vi "Main.vi"() -> ()   [LabVIEW 2025]
uses:
  TypeDefs/MainState.ctl
  random-number-analyzer-bak/Source/Typedefs/State_enum.ctl
  <vilib>/Analysis/baseanly.llb/Mean (DBL).vi
  <vilib>/Analysis/NI_AALBase.lvlib
  Utilities/Random/Random.lvlib
panel:
  in  "Find Minimum":bool
  in  "Find Maximum":bool
  in  "Compute Average":bool
  in  "Generate Random":bool
  out "Waveform Graph":dbl[](graph)
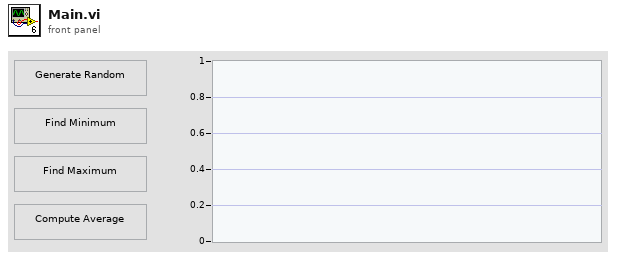
[diagram p1: front panel]
types:
  T1 = typedef "MainState.ctl" = enum16{"CONSTRUCT", "DESTRUCT", "WAITING_FOR_EVENT", "GENERATE_RANDOM", "FIND_MINIMUM", "FIND_MAXIMUM", "COMPUTE_AVERAGE"}
  T2 = typedef "State_enum.ctl" = enum16{"CONSTRUCT", "DESTRUCT", "WAITING_FOR_EVENT", "GENERATE_RANDOM", "FIND_MINIMUM", "FIND_MAXIMUM", "COMPUTE_AVERAGE"}
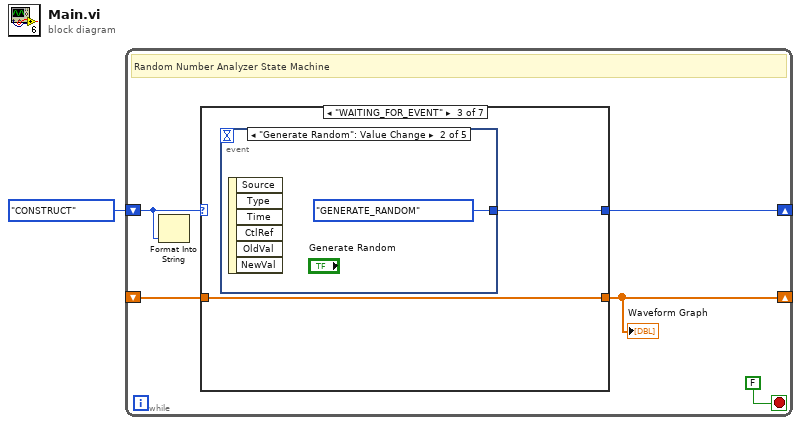
[diagram p0: block diagram]
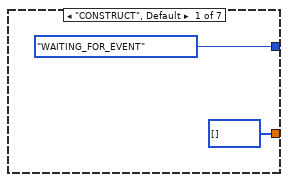
[diagram p2: hidden frame]
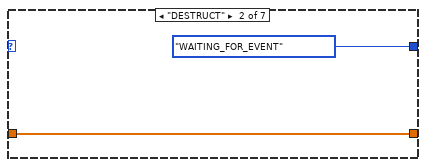
[diagram p3: hidden frame]
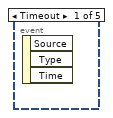
[diagram p4: hidden frame]
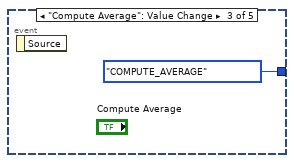
[diagram p5: hidden frame]
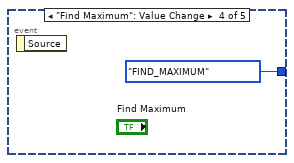
[diagram p6: hidden frame]
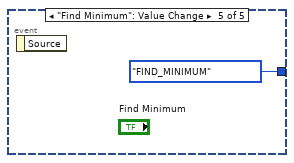
[diagram p7: hidden frame]
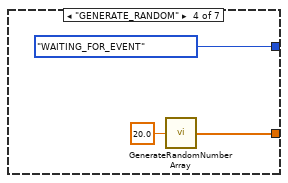
[diagram p8: hidden frame]
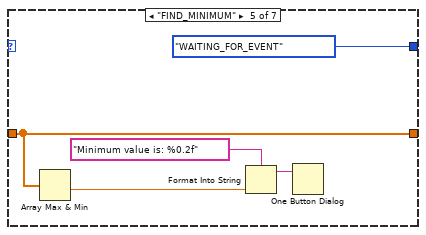
[diagram p9: hidden frame]
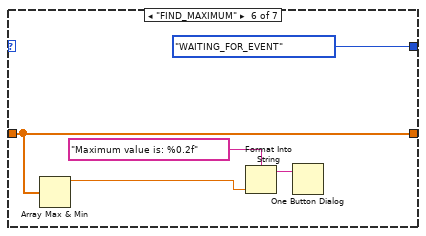
[diagram p10: hidden frame]
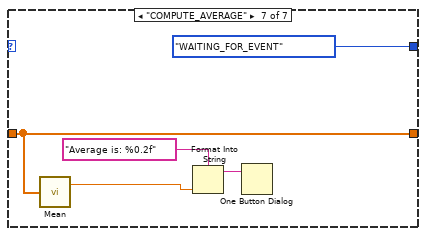
[diagram p11: hidden frame]
diagram:
  n1 = while {
    shift-right: [w5] -> _
    shift-left: MainState."CONSTRUCT" -> [w4]
    shift-right: [w2] -> _
    shift-left: _ -> [w3]
    stop <- FALSE stop-if-true
    # "Random Number Analyzer State Machine"
    n2 = Format Into String(w4) -> ()  [unwired: 3 in, 2 out]
    n3 = case shown="\"WAITING_FOR_EVENT\"" w4 {
      tunnel: [MainState."WAITING_FOR_EVENT" MainState."WAITING_FOR_EVENT" w11 MainState."WAITING_FOR_EVENT" MainState."WAITING_FOR_EVENT" MainState."WAITING_FOR_EVENT" MainState."WAITING_FOR_EVENT"] -> w5
      tunnel: [i32[] [] w10 w12 w17 w23 w25 w33] -> w2
      tunnel: w3 -> [_ w10 w12 _ w23 w25 w33]
      frame "CONSTRUCT", Default {
      }
      frame "DESTRUCT" {
      }
      frame "WAITING_FOR_EVENT" {
        n4 = event shown="[1] \"Generate Random\": Value Change" {
          selector: _ -> [_ _ _ _ _]
          dyn-events: _ -> [_ _ _ _ _]
          timeout: _ -> [_ _ _ _ _]
          tunnel: [_ MainState."GENERATE_RANDOM" State_enum."COMPUTE_AVERAGE" State_enum."FIND_MAXIMUM" State_enum."FIND_MINIMUM"] -> w11
          event Timeout {
            n5 = event-data() -> ()  [unwired: 1 in, 3 out]
          }
          event "Generate Random": Value Change {
            n6 = event-data() -> ()  [unwired: 1 in, 6 out]
          }
          event "Compute Average": Value Change {
            n7 = event-data() -> ()  [unwired: 1 in, 1 out]
          }
          event "Find Maximum": Value Change {
            n8 = event-data() -> ()  [unwired: 1 in, 1 out]
          }
          event "Find Minimum": Value Change {
            n9 = event-data() -> ()  [unwired: 1 in, 1 out]
          }
        }
      }
      frame "GENERATE_RANDOM" {
        n10 = call "GenerateRandomNumberArray.vi"("Size"=20.0) -> ("Array"=w17:dbl[])
      }
      frame "FIND_MINIMUM" {
        n11 = Array Max & Min(array=w23) -> (min value=w20:dbl)  [unwired: 3 out]
        n12 = Format Into String(format string="Minimum value is: %0.2f", w20) -> (resulting string=w21:string)  [unwired: 2 in, 1 out]
        n13 = One Button Dialog(message=w21) -> ()  [unwired: 1 in, 1 out]
      }
      frame "FIND_MAXIMUM" {
        n14 = Array Max & Min(array=w25) -> (max value=w28:dbl)  [unwired: 3 out]
        n15 = Format Into String(format string="Maximum value is: %0.2f", w28) -> (resulting string=w26:string)  [unwired: 2 in, 1 out]
        n16 = One Button Dialog(message=w26) -> ()  [unwired: 1 in, 1 out]
      }
      frame "COMPUTE_AVERAGE" {
        n17 = call-poly <vilib>:"Mean.vi"("X"=w33) -> ("mean"=w30:dbl)  [unwired: 1 out]
        n18 = Format Into String(format string="Average is: %0.2f", w30) -> (resulting string=w32:string)  [unwired: 2 in, 1 out]
        n19 = One Button Dialog(message=w32) -> ()  [unwired: 1 in, 1 out]
      }
    }
    "Waveform Graph" <- w2
  }
